vi "Tokenize.vi"(5 "delimiters (\\s,\\t,\\r,\\n,=)":string=" \t\r\n=", 6 "offset":i32, 7 "input string":string="ChargingState=CHARGE_OFF-0\r\nChargeWarning=NO\r\nTemperatureLevel=1\r\nIPG_ReceivedLevel=1") -> (1 "tokens":string[](array[string]), 2 "offset past token":i32=-1, 3 "string out":string)   [LabVIEW 2020]
doc: "Scans the input string, starting at offset, for tokens, and outputs an array of 32-bit integers."
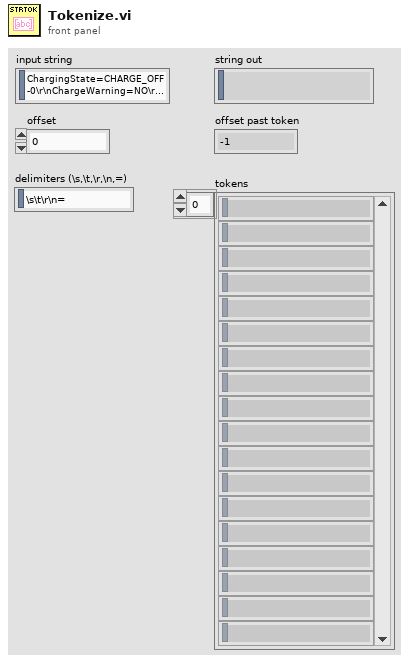
[diagram p1: front panel]
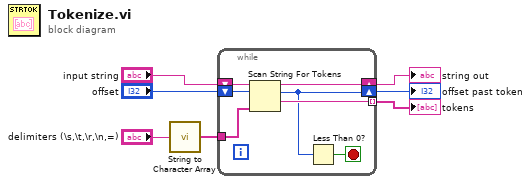
[diagram p0: block diagram]
diagram:
  n1 = call "String to Character Array.vi"("input string"="delimiters (\\s,\\t,\\r,\\n,=)") -> ("character array"=w6:string[])
  n2 = while {
    tunnel: w6 -> [w13]
    shift-right: [w12] -> w3
    shift-left: "input string" -> [w14]
    shift-right: [w8] -> w2
    shift-left: "offset" -> [w11]
    tunnel: [w10] -> w1 mode=indexing
    stop <- w9 stop-if-true
    n3 = Scan String For Tokens(6:w13, 8:w11, 9:w14) -> (1:w10:string, 2:w8:i32, 3:w12:string)  [unwired: 3 in, 1 out]
    n4 = Less Than 0?(x=w8) -> (x < 0?=w9:bool)
  }
  "string out" <- w3
  "offset past token" <- w2
  "tokens" <- w1
